vi "UpdateFPGARef.vi"(8 "error in (no error)":errorcluster, 10 "FPGA Target Main VI":string="nirviOpenFPGA", 11 "VI Refnum":refnum<vi>) -> (0 "error out":errorcluster, 3 "VI Refnum Out":refnum<vi>)   [LabVIEW 2021, in "myRIOMetaDataObj.lvclass"]
uses:
  myRIOMetaDataObj.lvclass
  <vilib>/Utility/traverseref.llb/TRef TravTarget.ctl
  <vilib>/rvi/ClientSDK/Core/Script/FpgaInterface/OpenFpgaVI/Private/GetVIConfiguration.vi
  <vilib>/rvi/ClientSDK/Core/Script/FpgaInterface/OpenFpgaVI/Private/SetVIConfiguration.vi
  <vilib>/rvi/ClientSDK/Core/Script/FpgaInterface/OpenFpgaVI/Private/niFpgaInterfaceXnApi_OpenFpgaVI.lvclass
  <vilib>/Utility/traverseref.llb/VI Scripting - Traverse.lvlib
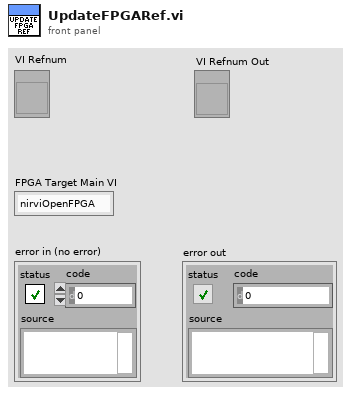
[diagram p1: front panel]
types:
  T1 = typedef "TRef TravTarget.ctl" = enum16{"FP", "BD", "Other"}
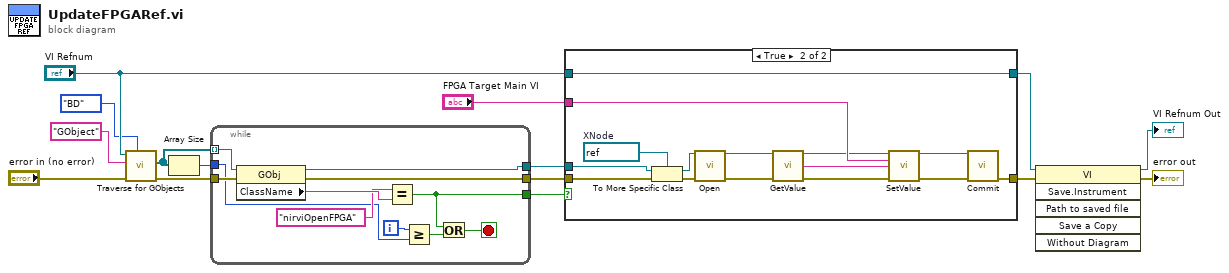
[diagram p0: block diagram]
diagram:
  n1 = call <vilib>:"Traverse for GObjects.vi"("Traverse Target"=TRef_TravTarget."BD", "error in (no error)"="error in (no error)", "Class Name"="GObject", "VI Refnum"="VI Refnum") -> ("error out"=w13:errorcluster, "References"=w12:refnum<vi>[])  [unwired: 4 in, 2 out]
  n2 = Array Size(array=w12) -> (size(s)=w11:i32)
  n3 = while {
    tunnel: w13 -> [w25]
    tunnel: w12 -> [w26] mode=indexing
    tunnel: [w24] -> w8
    tunnel: w11 -> [w20]
    tunnel: [w17] -> w10
    tunnel: [w16] -> w9
    i -> [w21]
    stop <- w19 stop-if-true
    n4 = property class="GObj"(reference=w26, error in=w25) -> (reference out=w16:refnum<vi>, error out=w24:errorcluster, "ClassName"=w23:string)
    n5 = Equal?(x="nirviOpenFPGA", y=w23) -> (x = y?=w17:bool)
    n6 = Greater Or Equal?(x=w21, y=w20) -> (x >= y?=w18:bool)
    n7 = Or(x=w17, y=w18) -> (x .or. y?=w19:bool)
  }
  n8 = case shown="True" w10 {
    tunnel: w9 -> [_ w42]
    tunnel: w8 -> [w28 w43]
    tunnel: "FPGA Target Main VI" -> [_ w40]
    tunnel: "VI Refnum" -> [w27 w31]
    tunnel: [w28 w32] -> w3
    tunnel: [w27 w31] -> w5
    frame False {
    }
    frame True {
      w30 = refnum<vi> refnum  # XNode
      n9 = To More Specific Class(target class=w30, reference=w42, error in=w43) -> (specific class reference=w29:refnum<vi>, error out=w41:errorcluster)
      n10 = call <vilib>:"Open.vi"("xnode reference"=w29, "error in (no error)"=w41) -> ("openFpgaVI out"=w39:refnum<class "niFpgaInterfaceXnApi_OpenFpgaVI.lvclass">, "error out"=w38:errorcluster)  [unwired: 12 in]
      n11 = call-poly <vilib>:"GetValue.vi"("openFpgaVI in"=w39, "error in (no error)"=w38) -> ("openFpgaVI out"=w36:refnum<class "niFpgaInterfaceXnApi_OpenFpgaVI.lvclass">, "target name"=w35:string, "error out"=w37:errorcluster)  [unwired: 10 in, 1 out]
      n12 = call-poly <vilib>:"SetValue.vi"("openFpgaVI in"=w36, "qualified VI name"=w40, "target name"=w35, "error in (no error)"=w37) -> ("openFpgaVI out"=w33:refnum<class "niFpgaInterfaceXnApi_OpenFpgaVI.lvclass">, "error out"=w34:errorcluster)  [unwired: 10 in]
      n13 = call-dynamic "Commit.vi"("openFpgaVI in"=w33, "error in (no error)"=w34) -> ("error out"=w32:errorcluster)  [unwired: 12 in, 1 out]
    }
  }
  n14 = invoke class="VI" method="Save.Instrument"(reference=w5, error in=w3) -> (reference out=→"VI Refnum Out":refnum<vi>, error out=→"error out":errorcluster)  [unwired: 4 in, 4 out]
